vi "INDEX - Tree Control.vi"() -> ()   [LabVIEW 2014]
panel:
  in  "Expand":bool
  in  "Collapse":bool
  in  "Delete all":bool
  in  "Save":bool
  in  "Open":bool
  in  "stop":bool
  in  "Remove":bool
  in  "Modify":bool
  in  "Add Child":bool
  in  "Add Parent":bool
  in  "Item(s)":string
  in  "Tree":string(tree)
  # "Command Editor"
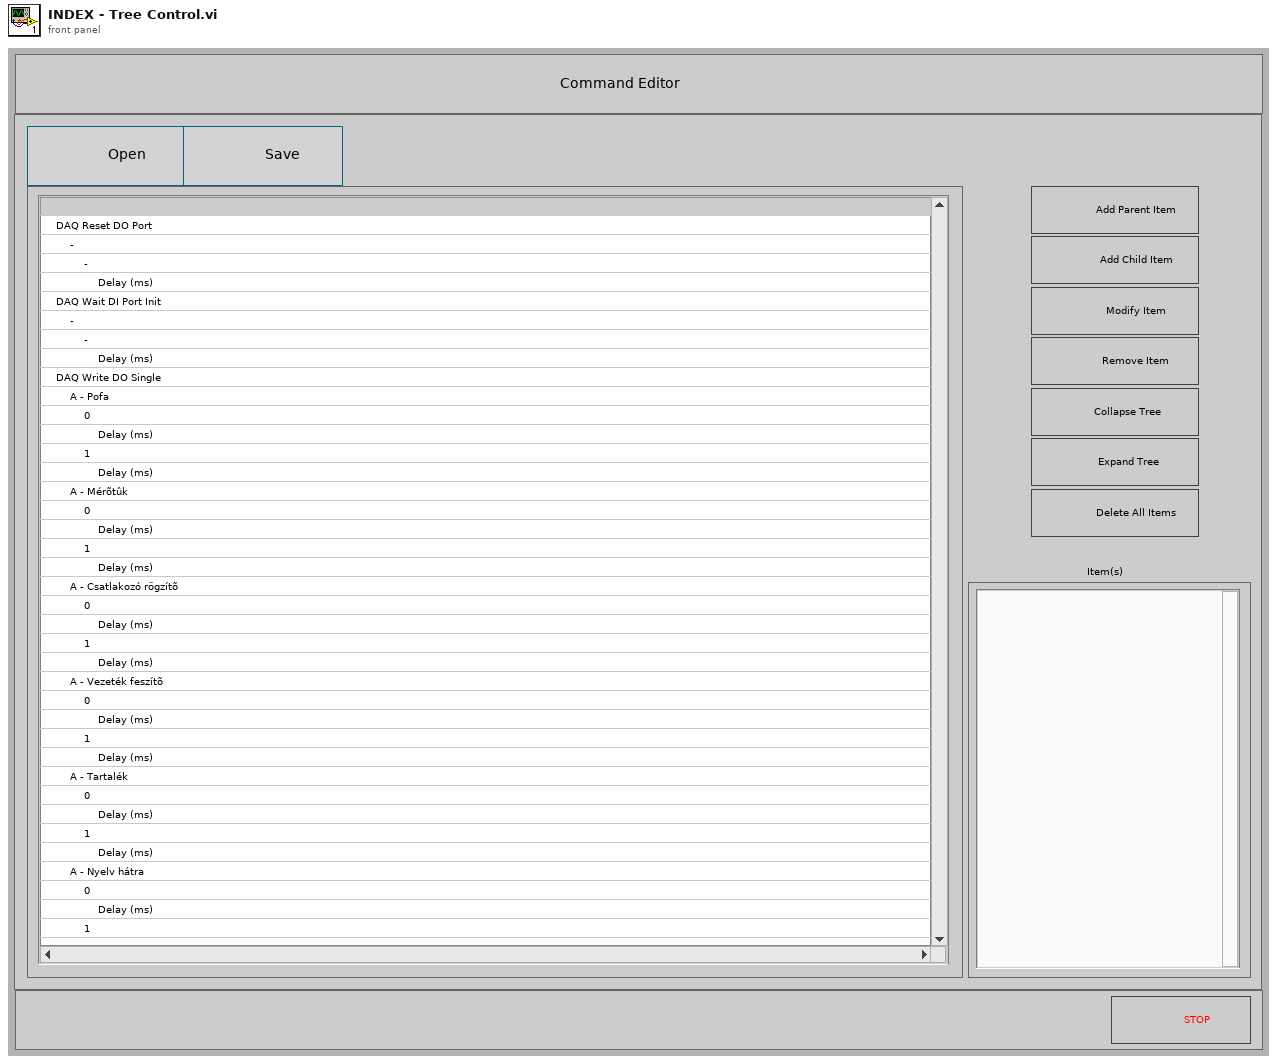
[diagram p1: front panel]
types:
  T1 = typedef "eventvkey.ctl" = enum16{"ASCII", "Enter", "Return", "Shift", "Ctrl", "Alt", "Cmd", "Opt", "Caps", "NumLock", "Clear", "Break", "Up", "Down", "Left", "Right", "Insert", "Delete", "Home", "End", "PageUp", "PageDown", "Escape", "Help", "Pause", "ScrollLock", "F1", "F2", "F3", "F4", "F5", "F6", "F7", "F8", "F9", "F10", "F11", "F12", "F13", "F14", "F15", "F16", "F17", "F18", "F19", "F20", "F21", "F22", "F23", "F24", "Play", "VolumeUp", "VolumeDown", "Mute", "Two Byte Char"}
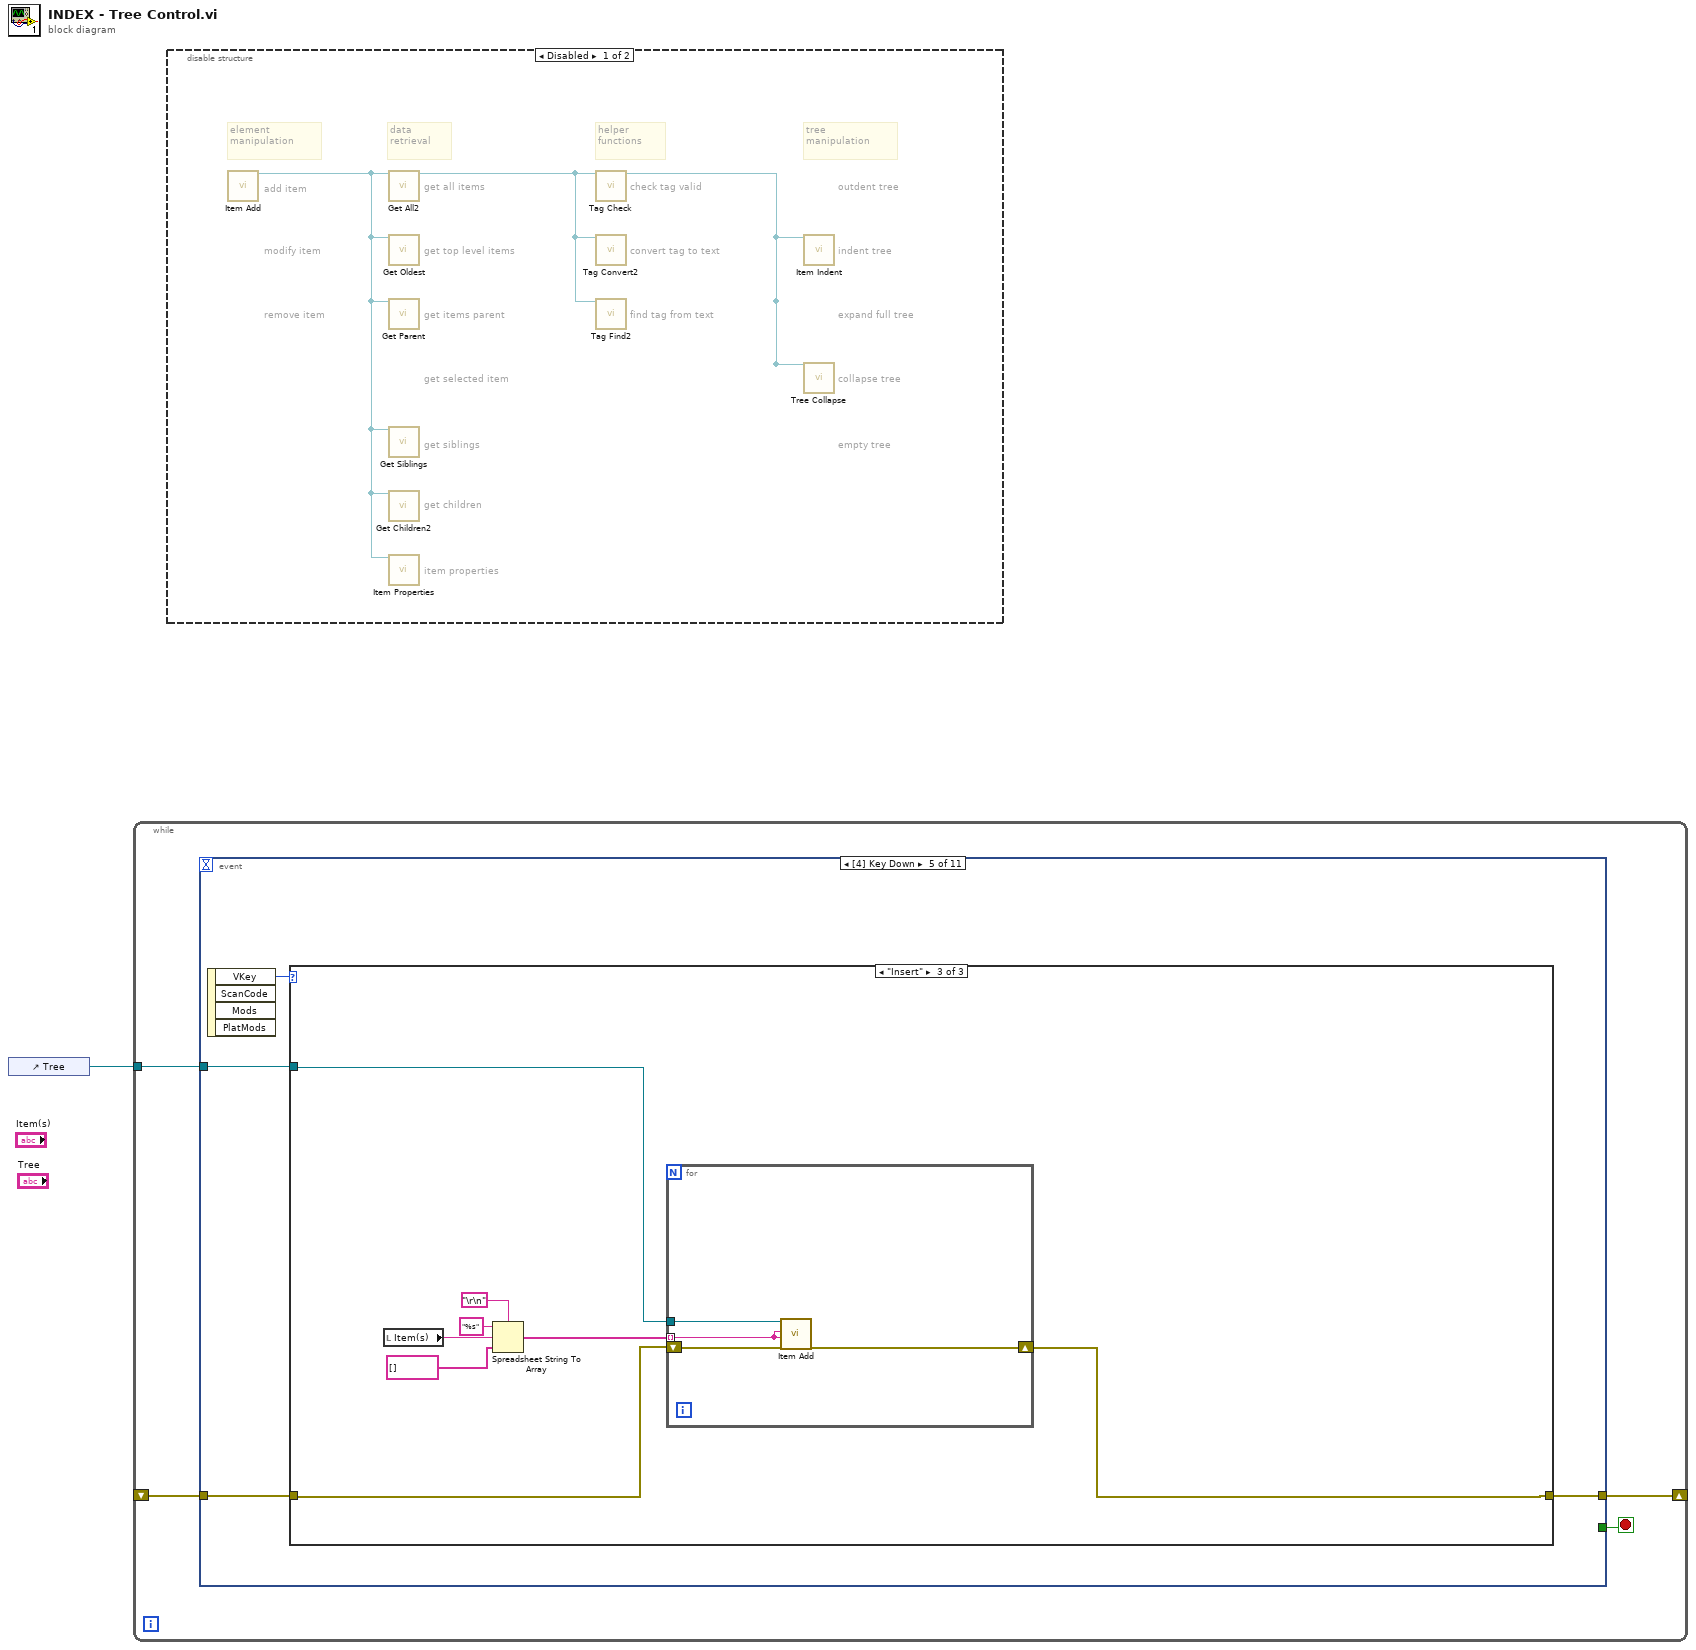
[diagram p0: block diagram]
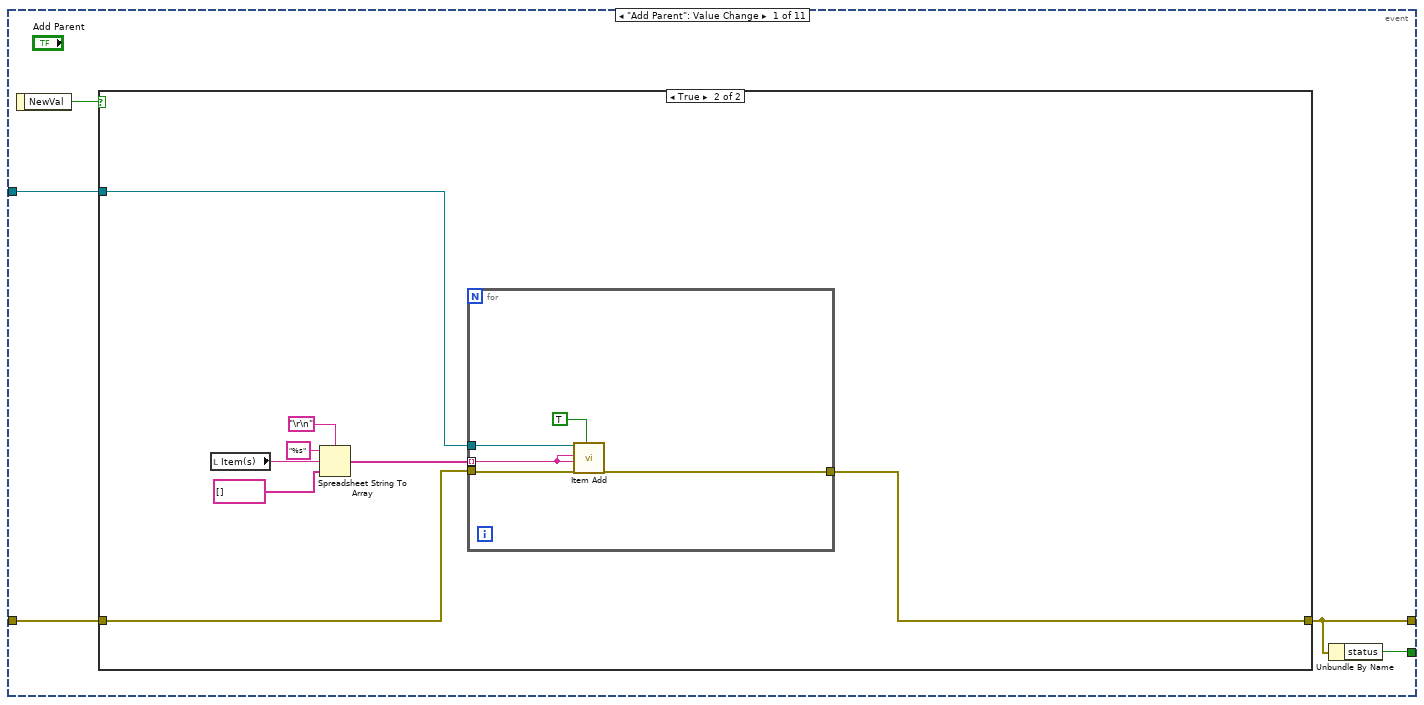
[diagram p2: hidden frame]
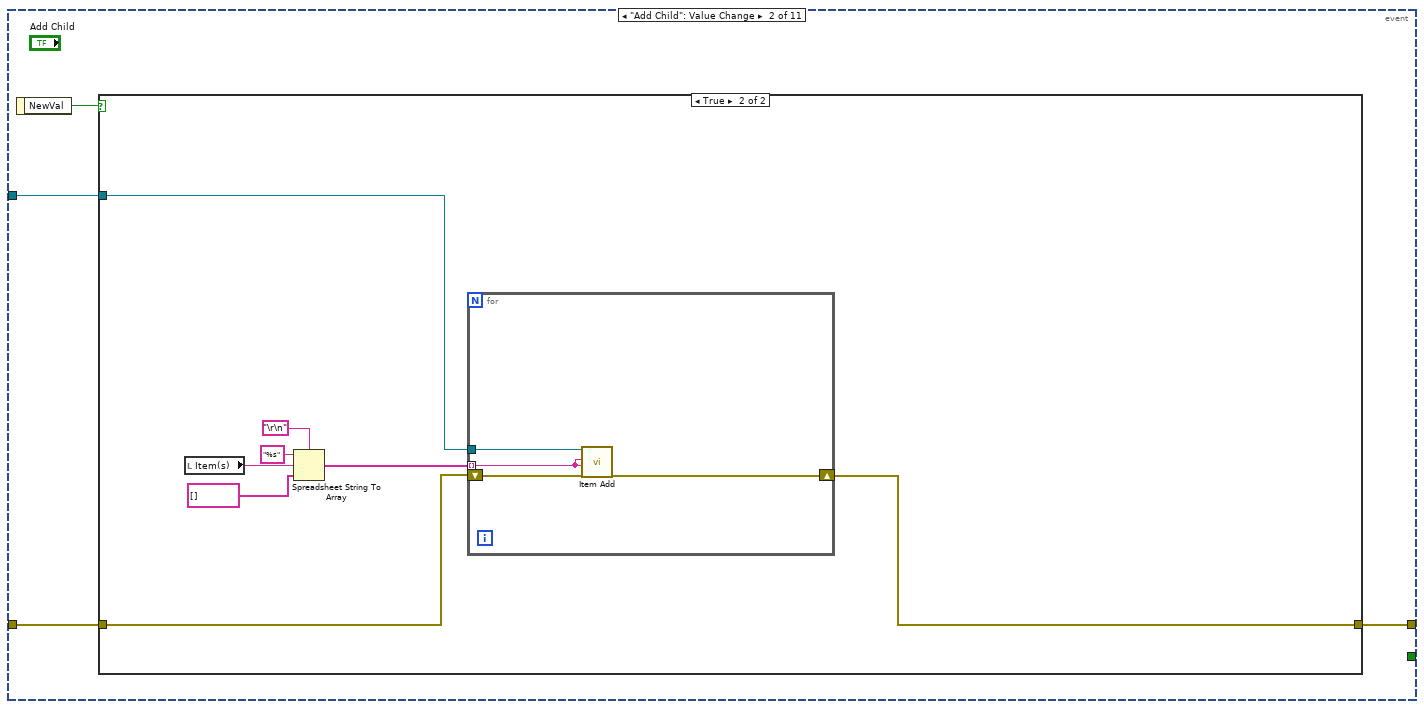
[diagram p4: hidden frame]
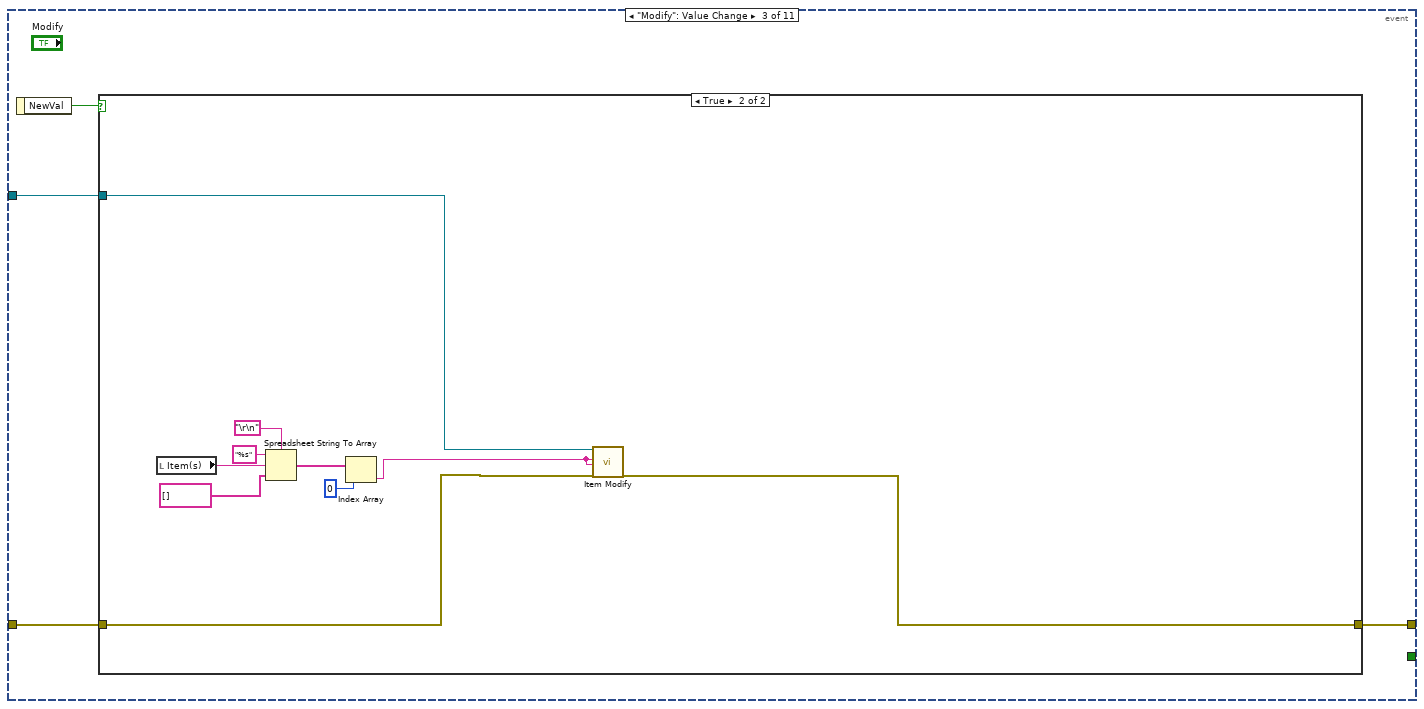
[diagram p6: hidden frame]
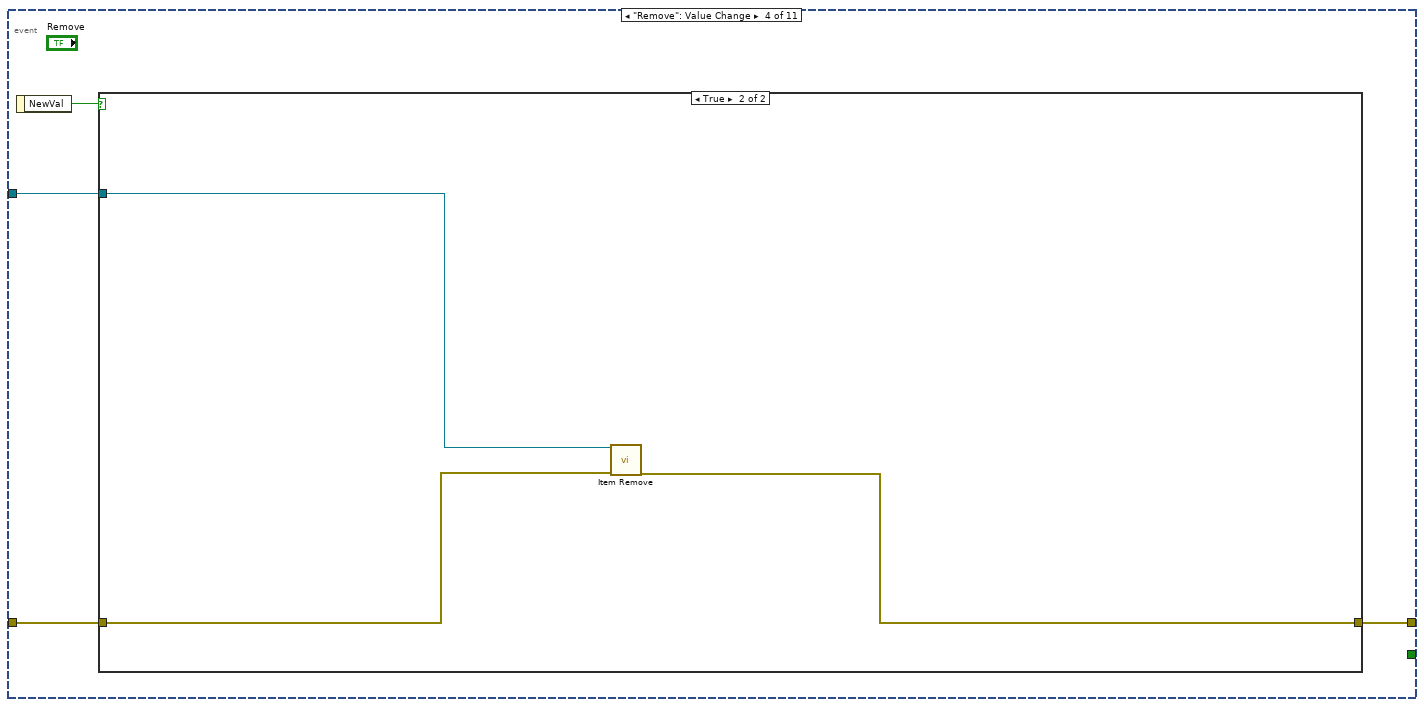
[diagram p8: hidden frame]
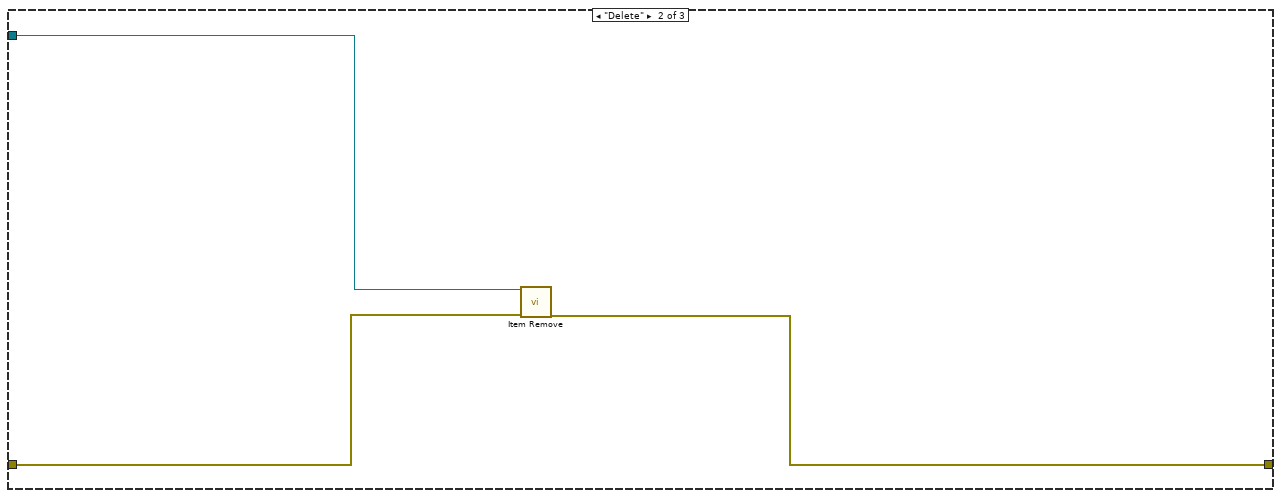
[diagram p11: hidden frame]
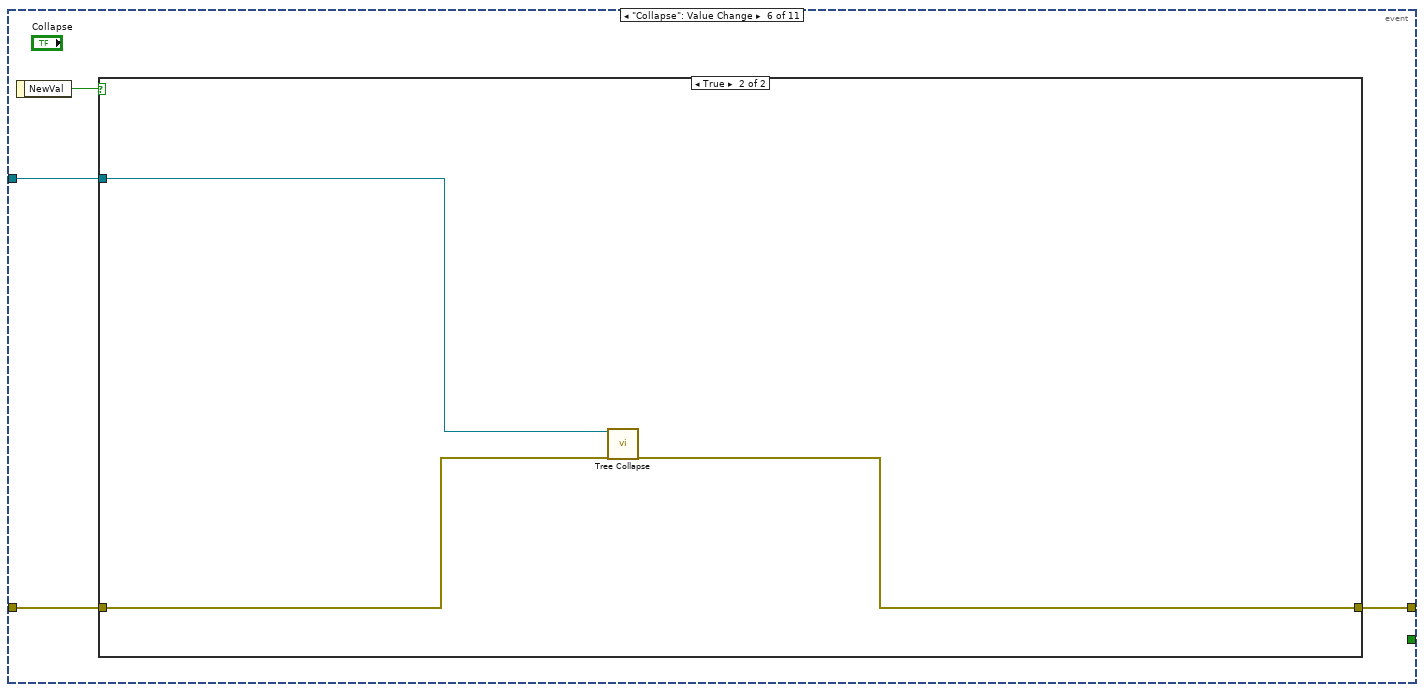
[diagram p12: hidden frame]
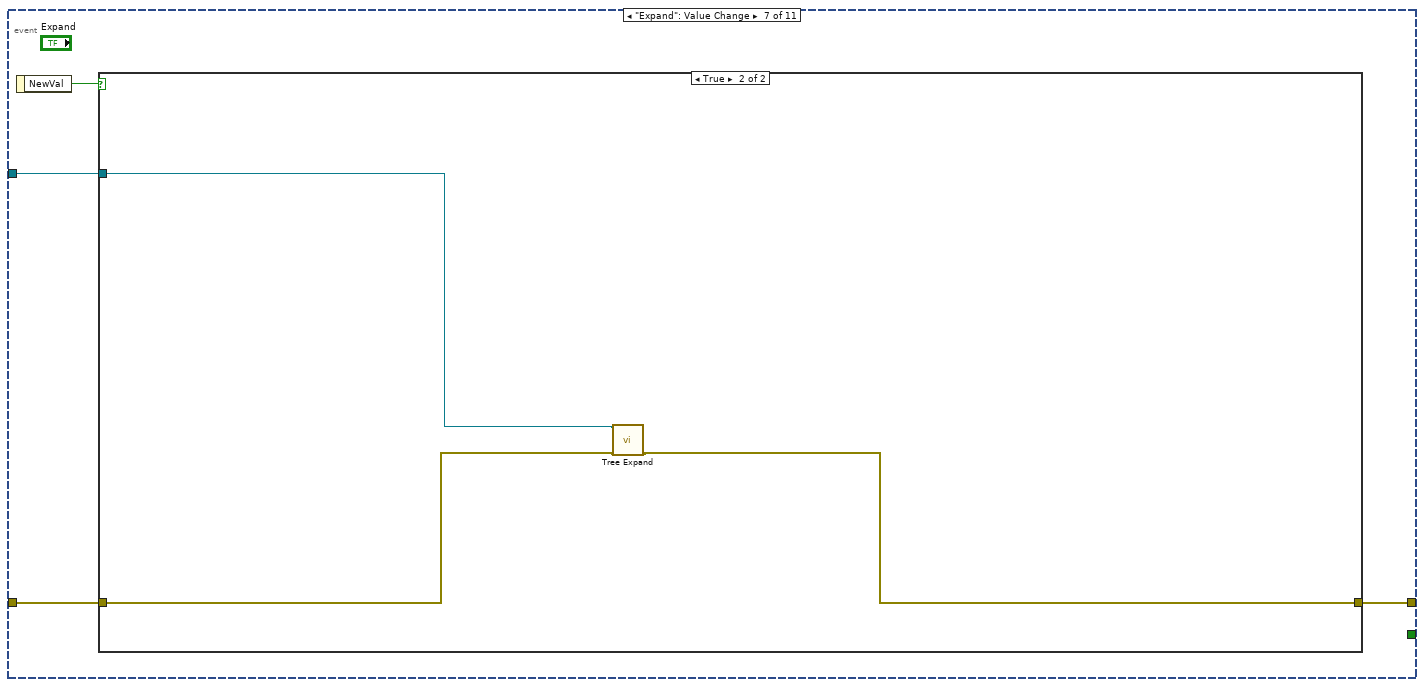
[diagram p14: hidden frame]
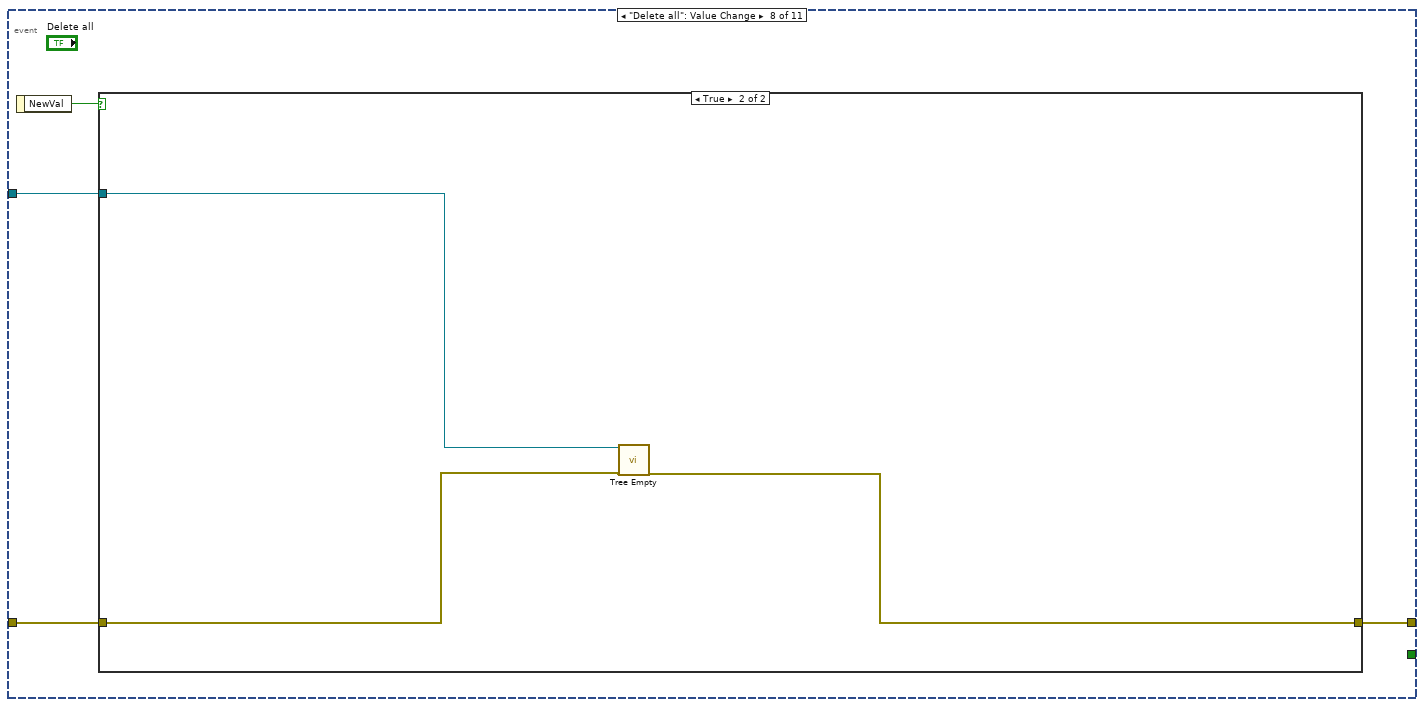
[diagram p16: hidden frame]
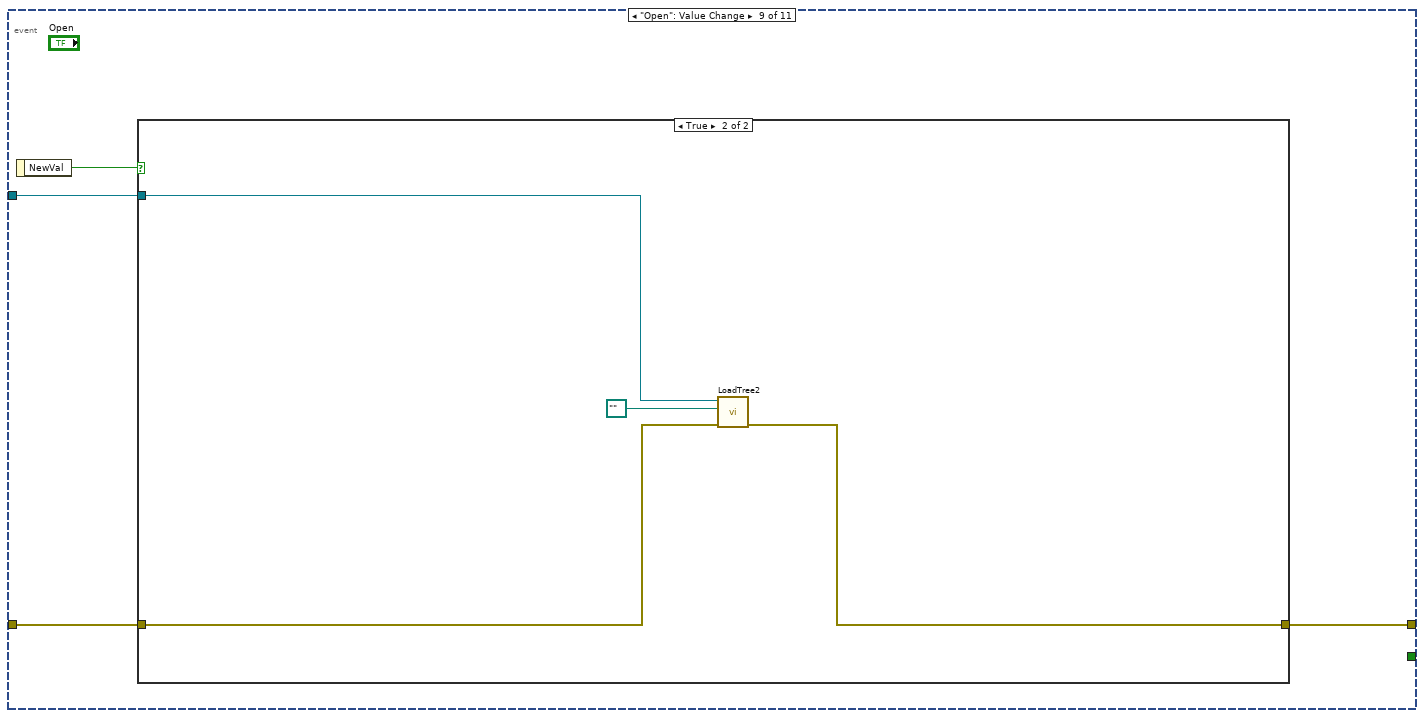
[diagram p18: hidden frame]
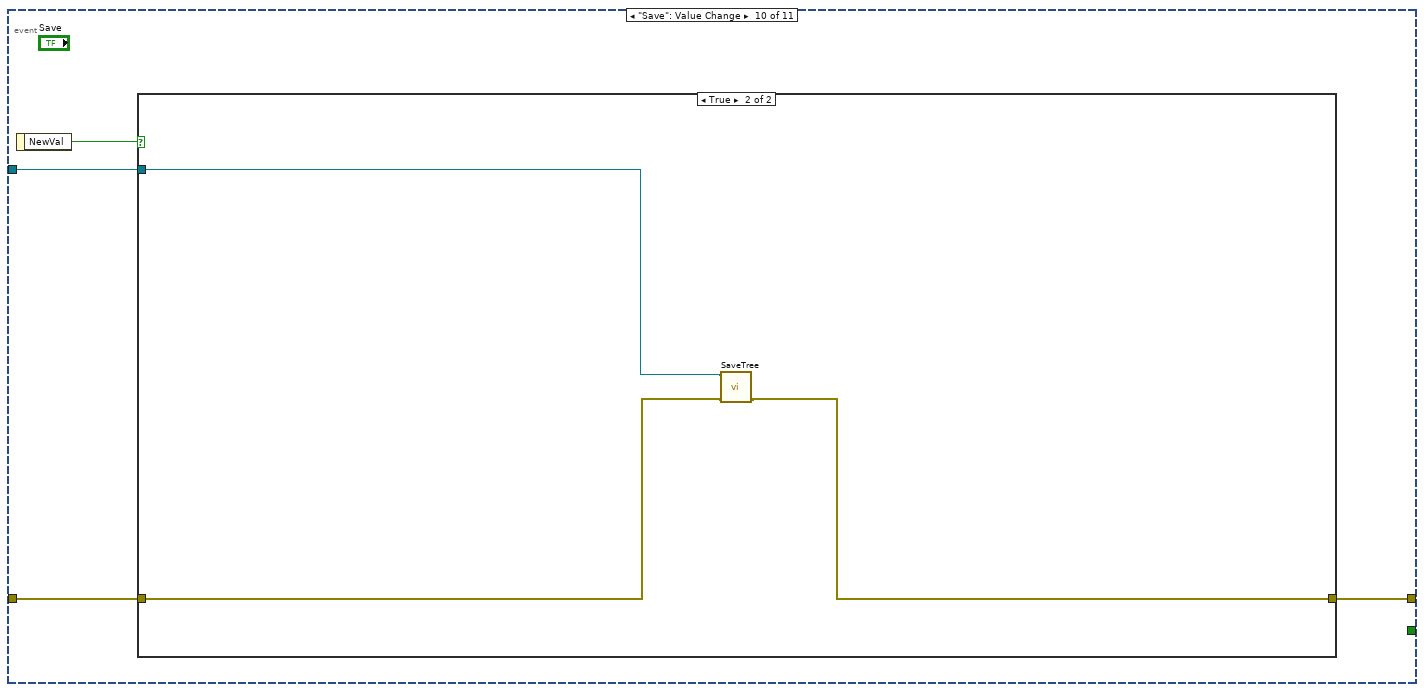
[diagram p20: hidden frame]
diagram:
  n1 = control-ref of="Tree"() -> (w1:refnum<vi>)
  n2 = while {
    shift-right: [w5] -> _
    shift-left: _ -> [w4]
    tunnel: w1 -> [w3]
    stop <- w2 stop-if-true
    n3 = event shown="[4] Key Down" {
      selector: _ -> [_ _ _ _ _ _ _ _ _ _ _]
      dyn-events: _ -> [_ _ _ _ _ _ _ _ _ _ _]
      timeout: _ -> [_ _ _ _ _ _ _ _ _ _ _]
      tunnel: [w7 w27 w44 w59 w67 w87 w95 w103 w110 w119 w127] -> w5
      tunnel: w4 -> [w9 w26 w43 w58 w66 w86 w94 w102 w111 w120 w128]
      tunnel: w3 -> [w8 w25 w42 w57 w65 w85 w93 w101 w109 w118 _]
      tunnel: [w6 _ _ _ _ _ _ _ _ _ w126] -> w2
      event "Add Parent": Value Change {
        n4 = event-data() -> ("NewVal"=w10:bool)  [unwired: 1 in]
        n5 = case shown="True" w10 {
          tunnel: [w11 w19] -> w7
          tunnel: w9 -> [w11 w18]
          tunnel: w8 -> [_ w12]
          frame False {
          }
          frame True {
            n6 = local read "Item(s)"() -> (w14:string)
            n7 = Spreadsheet String To Array(delimiter (Tab)="\r\n", format string="%s", spreadsheet string=w14, array type (2D Dbl)=string[] []) -> (array=w13:string[])
            n8 = for {
              tunnel: [w24] -> w19
              tunnel: w18 -> [w23]
              tunnel: w12 -> [w22]
              tunnel: w13 -> [w20] mode=indexing
              n9 = call "Item Add.vi"("Tree Reference In"=w22, "New Tag Value (Same as Text)"=w20, "New Text Value"=w20, "error in (no error)"=w23, "Make Top Level Item"=TRUE) -> ("error out"=w24:errorcluster)  [unwired: 12 in, 2 out]
            }
          }
        }
        n10 = Unbundle By Name(w7) -> ("status"=w6:bool)
      }
      event "Add Child": Value Change {
        n11 = event-data() -> ("NewVal"=w28:bool)  [unwired: 1 in]
        n12 = case shown="True" w28 {
          tunnel: [w29 w37] -> w27
          tunnel: w26 -> [w29 w36]
          tunnel: w25 -> [_ w30]
          frame False {
          }
          frame True {
            n13 = local read "Item(s)"() -> (w32:string)
            n14 = Spreadsheet String To Array(delimiter (Tab)="\r\n", format string="%s", spreadsheet string=w32, array type (2D Dbl)=string[] []) -> (array=w31:string[])
            n15 = for {
              tunnel: w30 -> [w39]
              tunnel: w31 -> [w38] mode=indexing
              shift-right: [w41] -> w37
              shift-left: w36 -> [w40]
              n16 = call "Item Add.vi"("Tree Reference In"=w39, "New Tag Value (Same as Text)"=w38, "New Text Value"=w38, "error in (no error)"=w40) -> ("error out"=w41:errorcluster)  [unwired: 13 in, 2 out]
            }
          }
        }
      }
      event "Modify": Value Change {
        n17 = event-data() -> ("NewVal"=w45:bool)  [unwired: 1 in]
        n18 = case shown="True" w45 {
          tunnel: [w46 w56] -> w44
          tunnel: w43 -> [w46 w55]
          tunnel: w42 -> [_ w50]
          frame False {
          }
          frame True {
            n19 = local read "Item(s)"() -> (w51:string)
            n20 = Spreadsheet String To Array(delimiter (Tab)="\r\n", format string="%s", spreadsheet string=w51, array type (2D Dbl)=string[] []) -> (array=w49:string[])
            n21 = Index Array(array=w49, index=0) -> (element=w47:string)
            n22 = call "Item Modify.vi"("Tree Reference In"=w50, "New Tag Value (No Change)"=w47, "New Text Value"=w47, "error in (no error)"=w55) -> ("error out"=w56:errorcluster)  [unwired: 14 in, 1 out]
          }
        }
      }
      event "Remove": Value Change {
        n23 = event-data() -> ("NewVal"=w60:bool)  [unwired: 1 in]
        n24 = case shown="True" w60 {
          tunnel: [w61 w62] -> w59
          tunnel: w58 -> [w61 w64]
          tunnel: w57 -> [_ w63]
          frame False {
          }
          frame True {
            n25 = call "Item Remove.vi"("Tree Reference In"=w63, "error in (no error)"=w64) -> ("error out"=w62:errorcluster)  [unwired: 16 in, 1 out]
          }
        }
      }
      event Key Down {
        n26 = event-data() -> ("VKey"=w68:T1)  [unwired: 1 in, 3 out]
        n27 = case shown="\"Insert\"" w68 {
          tunnel: [w69 w70 w75] -> w67
          tunnel: w66 -> [w69 w72 w74]
          tunnel: w65 -> [_ w71 w73]
          frame Default {
          }
          frame "Delete" {
            n28 = call "Item Remove.vi"("Tree Reference In"=w71, "error in (no error)"=w72) -> ("error out"=w70:errorcluster)  [unwired: 16 in, 1 out]
          }
          frame "Insert" {
            n29 = local read "Item(s)"() -> (w77:string)
            n30 = Spreadsheet String To Array(delimiter (Tab)="\r\n", format string="%s", spreadsheet string=w77, array type (2D Dbl)=string[] []) -> (array=w76:string[])
            n31 = for {
              tunnel: w73 -> [w82]
              tunnel: w76 -> [w81] mode=indexing
              shift-right: [w84] -> w75
              shift-left: w74 -> [w83]
              n32 = call "Item Add.vi"("Tree Reference In"=w82, "New Tag Value (Same as Text)"=w81, "New Text Value"=w81, "error in (no error)"=w83) -> ("error out"=w84:errorcluster)  [unwired: 13 in, 2 out]
            }
          }
        }
      }
      event "Collapse": Value Change {
        n33 = event-data() -> ("NewVal"=w88:bool)  [unwired: 1 in]
        n34 = case shown="True" w88 {
          tunnel: [w89 w90] -> w87
          tunnel: w86 -> [w89 w91]
          tunnel: w85 -> [_ w92]
          frame False {
          }
          frame True {
            n35 = call "Tree Collapse.vi"("Tree Reference In"=w92, "error in (no error)"=w91) -> ("error out"=w90:errorcluster)  [unwired: 16 in, 1 out]
          }
        }
      }
      event "Expand": Value Change {
        n36 = event-data() -> ("NewVal"=w96:bool)  [unwired: 1 in]
        n37 = case shown="True" w96 {
          tunnel: [w97 w99] -> w95
          tunnel: w94 -> [w97 w100]
          tunnel: w93 -> [_ w98]
          frame False {
          }
          frame True {
            n38 = call "Tree Expand.vi"("Tree Reference In"=w98, "error in (no error)"=w100) -> ("error out"=w99:errorcluster)  [unwired: 16 in, 1 out]
          }
        }
      }
      event "Delete all": Value Change {
        n39 = event-data() -> ("NewVal"=w104:bool)  [unwired: 1 in]
        n40 = case shown="True" w104 {
          tunnel: [w105 w106] -> w103
          tunnel: w102 -> [w105 w107]
          tunnel: w101 -> [_ w108]
          frame False {
          }
          frame True {
            n41 = call "Tree Empty.vi"("Tree Reference In"=w108, "error in (no error)"=w107) -> ("error out"=w106:errorcluster)  [unwired: 15 in, 2 out]
          }
        }
      }
      event "Open": Value Change {
        n42 = event-data() -> ("NewVal"=w112:bool)  [unwired: 1 in]
        n43 = case shown="True" w112 {
          tunnel: w111 -> [w113 w117]
          tunnel: [w113 w116] -> w110
          tunnel: w109 -> [_ w115]
          frame False {
          }
          frame True {
            n44 = call "LoadTree2.vi"("error in"=w117, "File Path Control"=path "", "TreeControl reference"=w115) -> ("error out"=w116:errorcluster)  [unwired: 8 in]
          }
        }
      }
      event "Save": Value Change {
        n45 = event-data() -> ("NewVal"=w121:bool)  [unwired: 1 in]
        n46 = case shown="True" w121 {
          tunnel: w120 -> [w122 w124]
          tunnel: [w122 w125] -> w119
          tunnel: w118 -> [_ w123]
          frame False {
          }
          frame True {
            n47 = call "SaveTree.vi"("error in"=w124, "TreeControl in"=w123) -> ("error out"=w125:errorcluster)  [unwired: 9 in]
          }
        }
      }
      event "stop": Value Change {
        n48 = event-data() -> ("NewVal"=w129:bool)  [unwired: 1 in]
        n49 = case shown="True" w129 {
          tunnel: w128 -> [w131 w133]
          tunnel: [w131 w133] -> w127
          tunnel: [FALSE TRUE] -> w126
          frame False {
          }
          frame True {
          }
        }
      }
    }
  }
  n50 = disable-structure shown="Disabled" {
    frame Disabled {
      # "empty tree"
      # "collapse tree"
      # "expand full tree"
      # "indent tree"
      # "outdent tree"
      # "find tag from text"
      # "convert tag to text"
      # "check tag valid"
      # "get children"
      # "get siblings"
      # "get selected item"
      # "get items parent"
      # "get top level items"
      # "get all items"
      # "item properties"
      # "remove item"
      # "modify item"
      # "add item"
      # "tree\nmanipulation"
      # "helper\nfunctions"
      # "data\nretrieval"
      # "element\nmanipulation"
      n51 = call "Item Add.vi"() -> ("Tree Reference Out"=w134:refnum<vi>)  [unwired: 17 in, 2 out]
      n52 = call "Get All2.vi"("Tree Reference In"=w134) -> ("Tree Reference Out"=w135:refnum<vi>)  [unwired: 15 in, 3 out]
      n53 = call "Get Oldest.vi"("Tree Reference In"=w134) -> ()  [unwired: 16 in, 3 out]
      n54 = call "Get Parent.vi"("Tree Reference In"=w134) -> ()  [unwired: 15 in, 4 out]
      n55 = call "Get Siblings.vi"("Tree Reference In"=w134) -> ()  [unwired: 16 in, 3 out]
      n56 = call "Get Children2.vi"("Tree Reference In"=w134) -> ()  [unwired: 16 in, 3 out]
      n57 = call "Item Properties.vi"("Tree Reference In"=w134) -> ()  [unwired: 13 in, 6 out]
      n58 = call "Tag Check.vi"("Tree Reference In"=w135) -> ("Tree Reference Out"=w136:refnum<vi>)  [unwired: 15 in, 3 out]
      n59 = call "Tag Convert2.vi"("Tree Reference In"=w135) -> ()  [unwired: 15 in, 4 out]
      n60 = call "Tag Find2.vi"("Tree Reference In"=w135) -> ()  [unwired: 15 in, 4 out]
      n61 = call "Item Indent.vi"("Tree Reference In"=w136) -> ()  [unwired: 17 in, 2 out]
      n62 = call "Tree Collapse.vi"("Tree Reference In"=w136) -> ()  [unwired: 17 in, 2 out]
    }
    frame Enabled {
    }
  }
